vi "view_without_raytrace.vi"(5 "offset":cluster{"x":i32, "y":i32}={"x"=100, "y"=100}, 6 "xy_angle_of light":dbl[](array[slide])=[1.4387755102040816, -7.979727989493313e-17] scale=-3.14..3.14, 7 "d-distance":dbl=0.004, 8 "Scens":T1(array[cluster]), 9 "new picture":picture) -> (3 "new picture 2":picture)   [LabVIEW 2011]
uses:
  <vilib>/Analysis/baseanly.llb/A x Vector.vi
  <vilib>/Analysis/NI_AALBase.lvlib
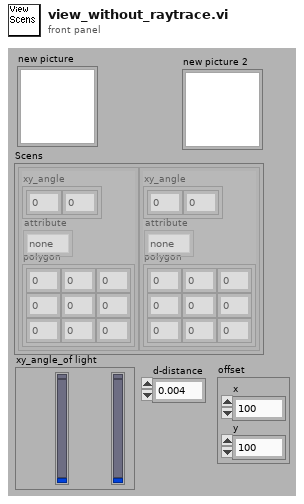
[diagram p1: front panel]
types:
  T1 = cluster{"xy_angle":dbl[], "polygon":dbl[][], "attribute":enum16{"none", "transparent", "reflective", "white", "black", "grey", "red", "yellow", "green", "blue", "pink"}}[]
  T2 = enum16{"none", "transparent", "reflective", "white", "black", "grey", "red", "yellow", "green", "blue", "pink"}
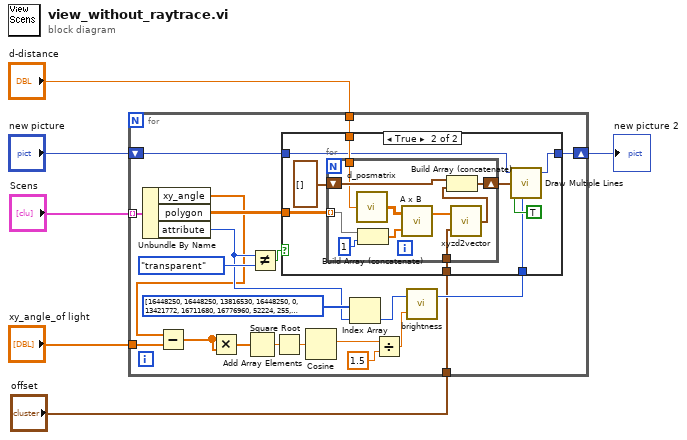
[diagram p0: block diagram]
diagram:
  n1 = for {
    tunnel: "Scens" -> [w27] mode=indexing
    tunnel: "d-distance" -> [w24]
    shift-right: [w22] -> w4
    shift-left: "new picture" -> [w23]
    tunnel: "xy_angle_of light" -> [w10]
    tunnel: "offset" -> [w9]
    n2 = Unbundle By Name(w27) -> ("xy_angle"=w11:dbl[], "polygon"=w26:dbl[][], "attribute"=w19:T2)
    n3 = Subtract(x=w11, y=w10) -> (x-y=w8:dbl[])
    n4 = Multiply(x=w8, y=w8) -> (x*y=w7:dbl[])
    n5 = Add Array Elements(numeric array=w7) -> (sum=w17:dbl)
    n6 = Not Equal?(x=w19, y=T2."transparent") -> (x != y?=w21:bool)
    n7 = Square Root(x=w17) -> (sqrt(x)=w16:dbl)
    n8 = Cosine(x=w16) -> (cos(x)=w14:dbl)
    n9 = Index Array(array=u32[] [16448250, 16448250, 13816530, 16448250, 0, 13421772, 16711680, 16776960, 52224, 255, 13369548], index=w19) -> (element=w18:u32)
    n10 = Divide(x=w14, y=1.5) -> (x/y=w12:dbl)
    n11 = call "brightness.vi"("brightness"=w12, "Colocr_in"=w18) -> ("Color_out"=w15:u32)  [unwired: 1 in]
    n12 = case shown="True" w21 {
      tunnel: w26 -> [_ w36]
      tunnel: w24 -> [_ w37]
      tunnel: [w28 w33] -> w22
      tunnel: w23 -> [w28 w32]
      tunnel: w15 -> [_ w30]
      tunnel: w9 -> [_ w29]
      frame False {
      }
      frame True {
        n13 = for {
          shift-right: [w47] -> w34
          shift-left: cluster{"x":i16, "y":i16}[] [] -> [w46]
          tunnel: w37 -> [w44]
          tunnel: w36 -> [w42] mode=indexing
          tunnel: w29 -> [w38]
          n14 = call "d_posmatrix.vi"("d-angle"=w44) -> ("d-matrix"=w45:dbl[][])
          n15 = Build Array (concatenate)(w42, 1) -> (w43:dbl[])
          n16 = call-poly <vilib>:"A x B.vi"("Vector"=w43, "A"=w45) -> ("A x Vector"=w40:dbl[])  [unwired: 1 out]
          n17 = call "xyzd2vector.vi"("offset"=w38, "xyzd"=w40) -> ("vector"=w39:cluster{"x":dbl, "y":dbl})
          n18 = Build Array (concatenate)(w46, w39) -> (w47:cluster{"x":dbl, "y":dbl}[])
        }
        n19 = call <vilib>:"Draw Multiple Lines.vi"("picture"=w32, "line endpoints"=w34, "fill?(F)"=TRUE, "color(black)"=w30) -> ("new picture"=w33:picture)  [unwired: 5 in]
      }
    }
  }
  "new picture 2" <- w4
